vi "Network Steam Read Connected.vi"(8 "error in (no error)":errorcluster, 11 "Model_AMC in":refnum<class "Model_AMC.lvclass">) -> (0 "error out":errorcluster, 2 "Connected?":bool, 3 "Model_AMC out":refnum<class "Model_AMC.lvclass">)   [LabVIEW 2021, in "Model_AMC.lvclass"]
uses:
  Model_AMC.lvclass
  Model_AMC.lvclass/Model_AMC.ctl
  <userlib>/John_Lib/Network_Streams_Connection/NetworkConnection.lvclass
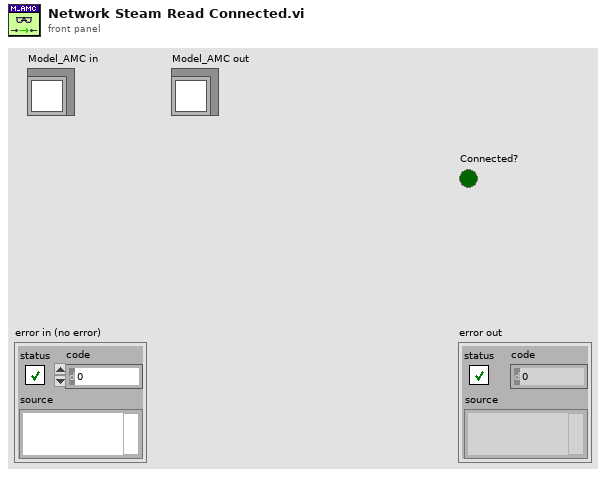
[diagram p1: front panel]
types:
  T1 = typedef "Model_AMC.lvclass/DVR.ctl" = cluster{"JKI_Network_Streams":refnum<class "NetworkConnection.lvclass">, "AMC Q":T2, "Connnected":bool}
  T2 = typedef "Model_AMC.lvclass/AMC Q.ctl" = cluster{"Main":T3, "OPCUA":T3, "NetworkSteam":T3}
  T3 = typedef "AMC_FW.lvlib/Queue.ctl" = cluster{"Q":T4, "Name":string}
  T4 = typedef "AMC_FW.lvlib/Message Queue.ctl" = refnum<queue>
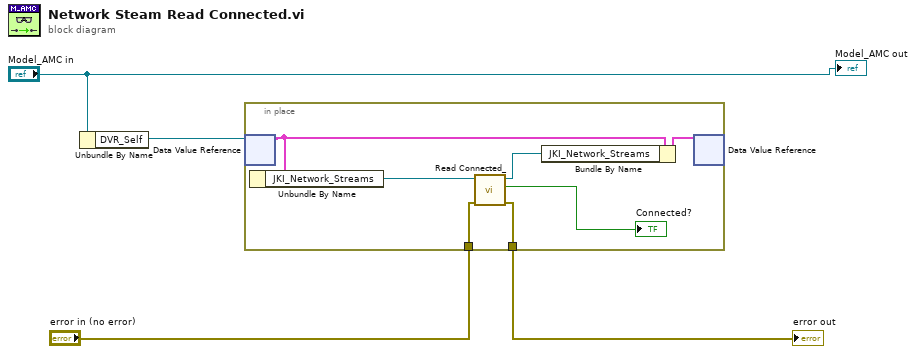
[diagram p0: block diagram]
diagram:
  n1 = Unbundle By Name("Model_AMC in") -> ("DVR_Self"=w4:refnum<data-value>)
  n2 = in-place {
    in-place-border: [w7] -> w3
    in-place-border: "error in (no error)" -> [w6]
    n3 = in-place-dvr #1(w4) -> (w11:T1)  [unwired: 1 out]
    n4 = Unbundle By Name(w11) -> ("JKI_Network_Streams"=w10:refnum<class "NetworkConnection.lvclass">)
    n5 = call <userlib>:"Read Connected_.vi"("error in (no error)"=w6, "NetworkConnection in"=w10) -> ("error out"=w7:errorcluster, "Connected?"=→"Connected?":bool, "NetworkConnection out"=w8:refnum<class "NetworkConnection.lvclass">)  [unwired: 7 in]
    n6 = Bundle By Name(cluster=w11, "JKI_Network_Streams"=w8) -> (w9:T1)
    n7 = in-place-dvr #1(w9) -> ()  [unwired: 2 out]
  }
  "error out" <- w3
  "Model_AMC out" <- "Model_AMC in"
